vi "New.vi"(8 "error in (no error)":errorcluster, 11 "reference in":refnum<class "DMM_Keysight_34980A.lvclass">) -> (0 "error out":errorcluster, 3 "reference out":refnum<class "DMM_Keysight_34980A.lvclass">)   [LabVIEW 2022 SP3, in "DMM_Keysight_34980A.lvlib" / "DMM_Keysight_34980A.lvclass"]
uses:
  DMM_Keysight_34980A.lvclass
  ObjectAttributes.ctl
  Config.ctl
  Mode.ctl
  DMM_Keysight_34980A.lvclass/DMM_Keysight_34980A.ctl
  Components/ViPER.lvlibp/ViPER.lvclass
panel:
  in  "Data":T1={"Config"={"VISA"=""}, "VISA ref"="", "Meas"=0.0, "Range DCV"=enum."Auto", "Range ACV"=enum."Default", "Range Ohms"=enum."Auto", "Range VFreq"=enum."Auto", " Range ACA"=enum."Auto", " Range DCA"=enum."Auto", "Mode"=enum."DCV", "Resolution"=enum."Default", "Bandwidth"=enum."20 Hz", "Low Frequency"=enum."20 Hz", "Aperture"=enum."100 ms", "Measurement"=[], "Time"=[], "Samples"=1, "dt"=0.0, "Timeout"=10000.0}
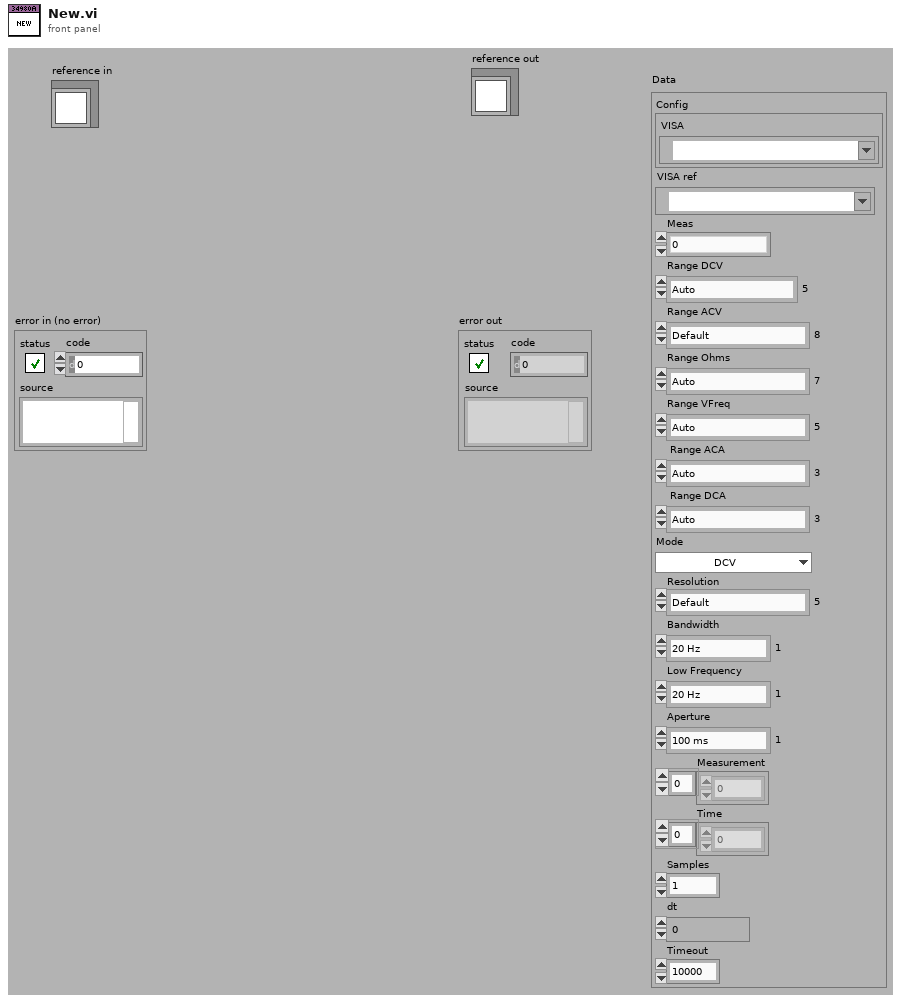
[diagram p1: front panel]
types:
  T1 = typedef "DMM_Keysight_34980A.lvlib/DMM_Keysight_34980A.lvclass/ObjectAttributes.ctl" = cluster{"Config":T2, "VISA ref":refnum<visa-resource-name>, "Meas":dbl, "Range DCV":enum16{"100 mV", "1 V", "10 V", "100 V", "300 V", "Auto", "Minimum", "Maximum"}, "Range ACV":enum16{"100 mV", "1 V", "10 V", "100 V", "300 V", "Auto", "Minimum", "Maximum", "Default"}, "Range Ohms":enum16{"100 Ohm", "1 kOhm", "10 kOhm", "100 kOhm", "1 MOhm", "10 MOhm", "100 MOhm", "Auto", "Minimum", "Maximum"}, "Range VFreq":enum16{"100 mV", "1 V", "10 V", "100 V", "300 V", "Auto", "Minimum", "Maximum"}, " Range ACA":enum16{"10 mA", "100 mA", "1 A", "Auto", "Minimum", "Maximum"}, " Range DCA":enum16{"10 mA", "100 mA", "1 A", "Auto", "Minimum", "Maximum"}, "Mode":T3, "Resolution":enum16{"4 1/2", "5 1/2", "6 1/2", "Least", "Highest", "Default"}, "Bandwidth":enum16{"3 Hz", "20 Hz", "200 Hz", "Minimum", "Maximum"}, "Low Frequency":enum16{"3 Hz", "20 Hz", "200 Hz", "Minimum", "Maximum"}, "Aperture":enum16{"10 ms", "100 ms", "1 sec", "Minimum", "Maximum"}, "Measurement":dbl[], "Time":dbl[], "Samples":u32, "dt":dbl, "Timeout":dbl}
  T2 = typedef "DMM_Keysight_34980A.lvlib/DMM_Keysight_34980A.lvclass/Config.ctl" = cluster{"VISA":refnum<visa-resource-name>}
  T3 = typedef "DMM_Keysight_34980A.lvlib/DMM_Keysight_34980A.lvclass/Mode.ctl" = enum16{"DCV", "ACV", "2W Ohms", "4W Ohms", "Frequency", "DCA", "ACA"}
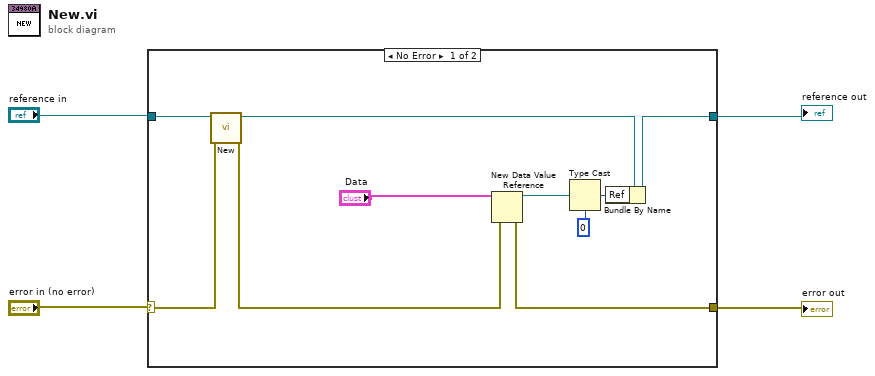
[diagram p0: block diagram]
diagram:
  n1 = case shown="No Error" "error in (no error)" {
    selector: "error in (no error)" -> [w6 w16]
    tunnel: [w7 w16] -> w2
    tunnel: "reference in" -> [w14 w15]
    tunnel: [w13 w15] -> w1
    frame No Error {
      n2 = call-parent "New.vi"("error in (no error)"=w6, "reference in"=w14) -> ("error out"=w5:errorcluster, "reference out"=w12:refnum<class "DMM_Keysight_34980A.lvclass">)  [unwired: 8 in]
      n3 = New Data Value Reference(data value="Data", error in=w5) -> (data value reference=w10:refnum<data-value>, error out=w7:errorcluster)
      n4 = Type Cast(type=u32 0 ("DataRef"), x=w10) -> (*(type *) &x=w9:u32)
      n5 = Bundle By Name(cluster=w12, "Ref"=w9) -> (w13:refnum<class "DMM_Keysight_34980A.lvclass">)
    }
    frame Error {
    }
  }
  "error out" <- w2
  "reference out" <- w1
